vi "HRM-AQN-myDAQ_init.vi"(11 "AQN cluster in":T1) -> (0 "error out":errorcluster, 3 "AQN cluster out":T1)   [LabVIEW 2020]
uses:
  HRM-AQN-input_clust.ctl
  <vilib>/DAQmx/create/channels.llb/DAQmx Create Channel (AI-Voltage-Basic).vi
  <vilib>/DAQmx/configure/timing.llb/DAQmx Timing (Sample Clock).vi
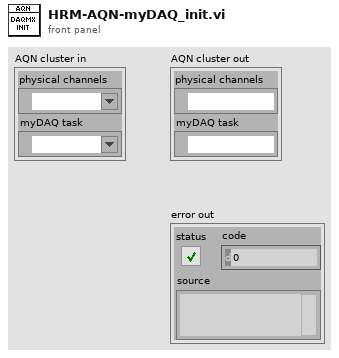
[diagram p1: front panel]
types:
  T1 = typedef "HRM-AQN-input_clust.ctl" = cluster{"physical channels":tag, "myDAQ task":refnum<k21>}
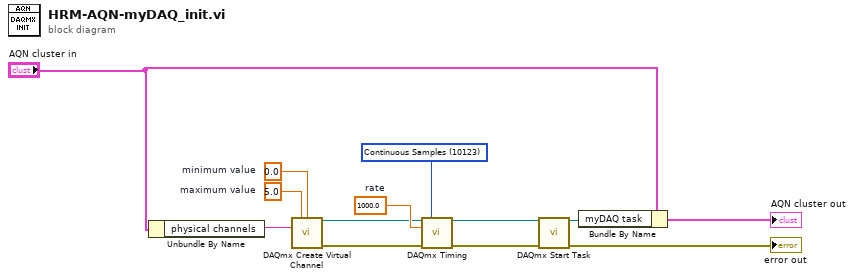
[diagram p0: block diagram]
diagram:
  w9 = 1000.0  # rate
  w8 = 10123 items=["Finite Samples"=10178, "Continuous Samples"=10123, "Hardware Timed Single Point"=12522] ("sample mode")
  w7 = 0.0  # minimum value
  w6 = 5.0  # maximum value
  n1 = Unbundle By Name("AQN cluster in") -> ("physical channels"=w10:tag)
  n2 = call-poly <vilib>:"DAQmx Create Virtual Channel.vi"("maximum value"=w6, "minimum value"=w7, "physical channels"=w10) -> ("task out"=w1:refnum<k21>, "error out"=w2:errorcluster)  [unwired: 11 in]
  n3 = call-poly <vilib>:"DAQmx Timing.vi"("task/channels in"=w1, "sample mode"=w8, "rate"=w9, "error in"=w2) -> ("task out"=w3:refnum<k21>, "error out"=w4:errorcluster)  [unwired: 10 in]
  n4 = call <vilib>:"DAQmx Start Task.vi"("task/channels in"=w3, "error in"=w4) -> ("task out"=w11:refnum<k21>, "error out"=→"error out":errorcluster)  [unwired: 12 in]
  n5 = Bundle By Name(cluster="AQN cluster in", "myDAQ task"=w11) -> (→"AQN cluster out":T1)
